vi "Write_Stats_Impedance_Meas.vi"(4 "Z Phase":dbl[](array[numeric]), 5 "|Z| Mag":dbl[](array[numeric]), 6 "Output Stats Cluster":T1, 7 "Compensation and Gain":T2={"Rg_Vmon"=5000.0, "Rg_Imon"=5000.0, "ESL_Cal"=2.5e-07, "ESR_Cal"=0.0, "Cp_Cal"=0.0, "Rp_Cal"=0.0, "Use Open/Short\nCompensation"=FALSE, "R_Shunt"=10000.0, "RLoad"=1000000000.0, "RLoad_Meas"=1000000000.0} {"RLoad_Meas" format="%#_6p"; "RLoad" format="%#_6p"}, 8 "Test Params Cluster":T3={"Test Freq. (Hz)"=0.0, "Output Signal Amplitude\nVolts Pk"=0.0, "Sampling Time (s)"=0.0, "Sampling Rate (Hz)"=0.0, "Output Channel"="Dev2/ao0", "Current Channel"="Dev2/ai0", "Voltage Channel"="Dev2/ai0", "Trigger Channel"="/Dev2/ao/StartTrigger", "Number of runs"=5}, 9 "Experiment Title":string="Experiment Title", 10 "File Name String":string="Test", 11 "Path":path=path "C:/Users/MPI/Documents/Test Saving Data") -> ()   [LabVIEW 2022 SP3]
panel:
  in  "Meta-Data Array":dbl[](array[numeric])=[1.0]
  out "TDMS path":path=path "C:/Users/MPI/Documents/Test Saving Data/2022_01_06_23_07_06_Test.tdms"
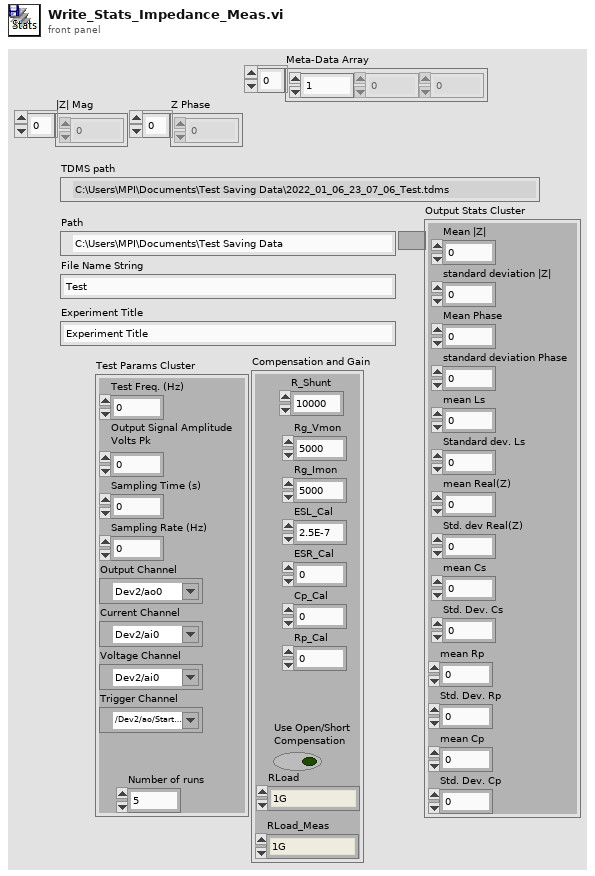
[diagram p1: front panel]
types:
  T1 = cluster{"Mean |Z|":dbl, "standard deviation |Z|":dbl, "Mean Phase":dbl, "standard deviation Phase":dbl, "mean Ls":dbl, "Standard dev. Ls":dbl, "mean Real(Z)":dbl, "Std. dev Real(Z)":dbl, "mean Cs":dbl, "Std. Dev. Cs":dbl, "Std. Dev. Rp":dbl, "mean Rp":dbl, "Std. Dev. Cp":dbl, "mean Cp":dbl}
  T2 = cluster{"Rg_Vmon":dbl, "Rg_Imon":dbl, "ESL_Cal":dbl, "ESR_Cal":dbl, "Cp_Cal":dbl, "Rp_Cal":dbl, "Use Open/Short\nCompensation":bool, "R_Shunt":dbl, "RLoad":dbl, "RLoad_Meas":dbl}
  T3 = cluster{"Test Freq. (Hz)":dbl, "Output Signal Amplitude\nVolts Pk":dbl, "Sampling Time (s)":dbl, "Sampling Rate (Hz)":dbl, "Output Channel":tag, "Current Channel":tag, "Voltage Channel":tag, "Trigger Channel":tag, "Number of runs":i32}
  T4 = enum16{"open", "open or create", "create or replace", "create", "open (read-only)"}
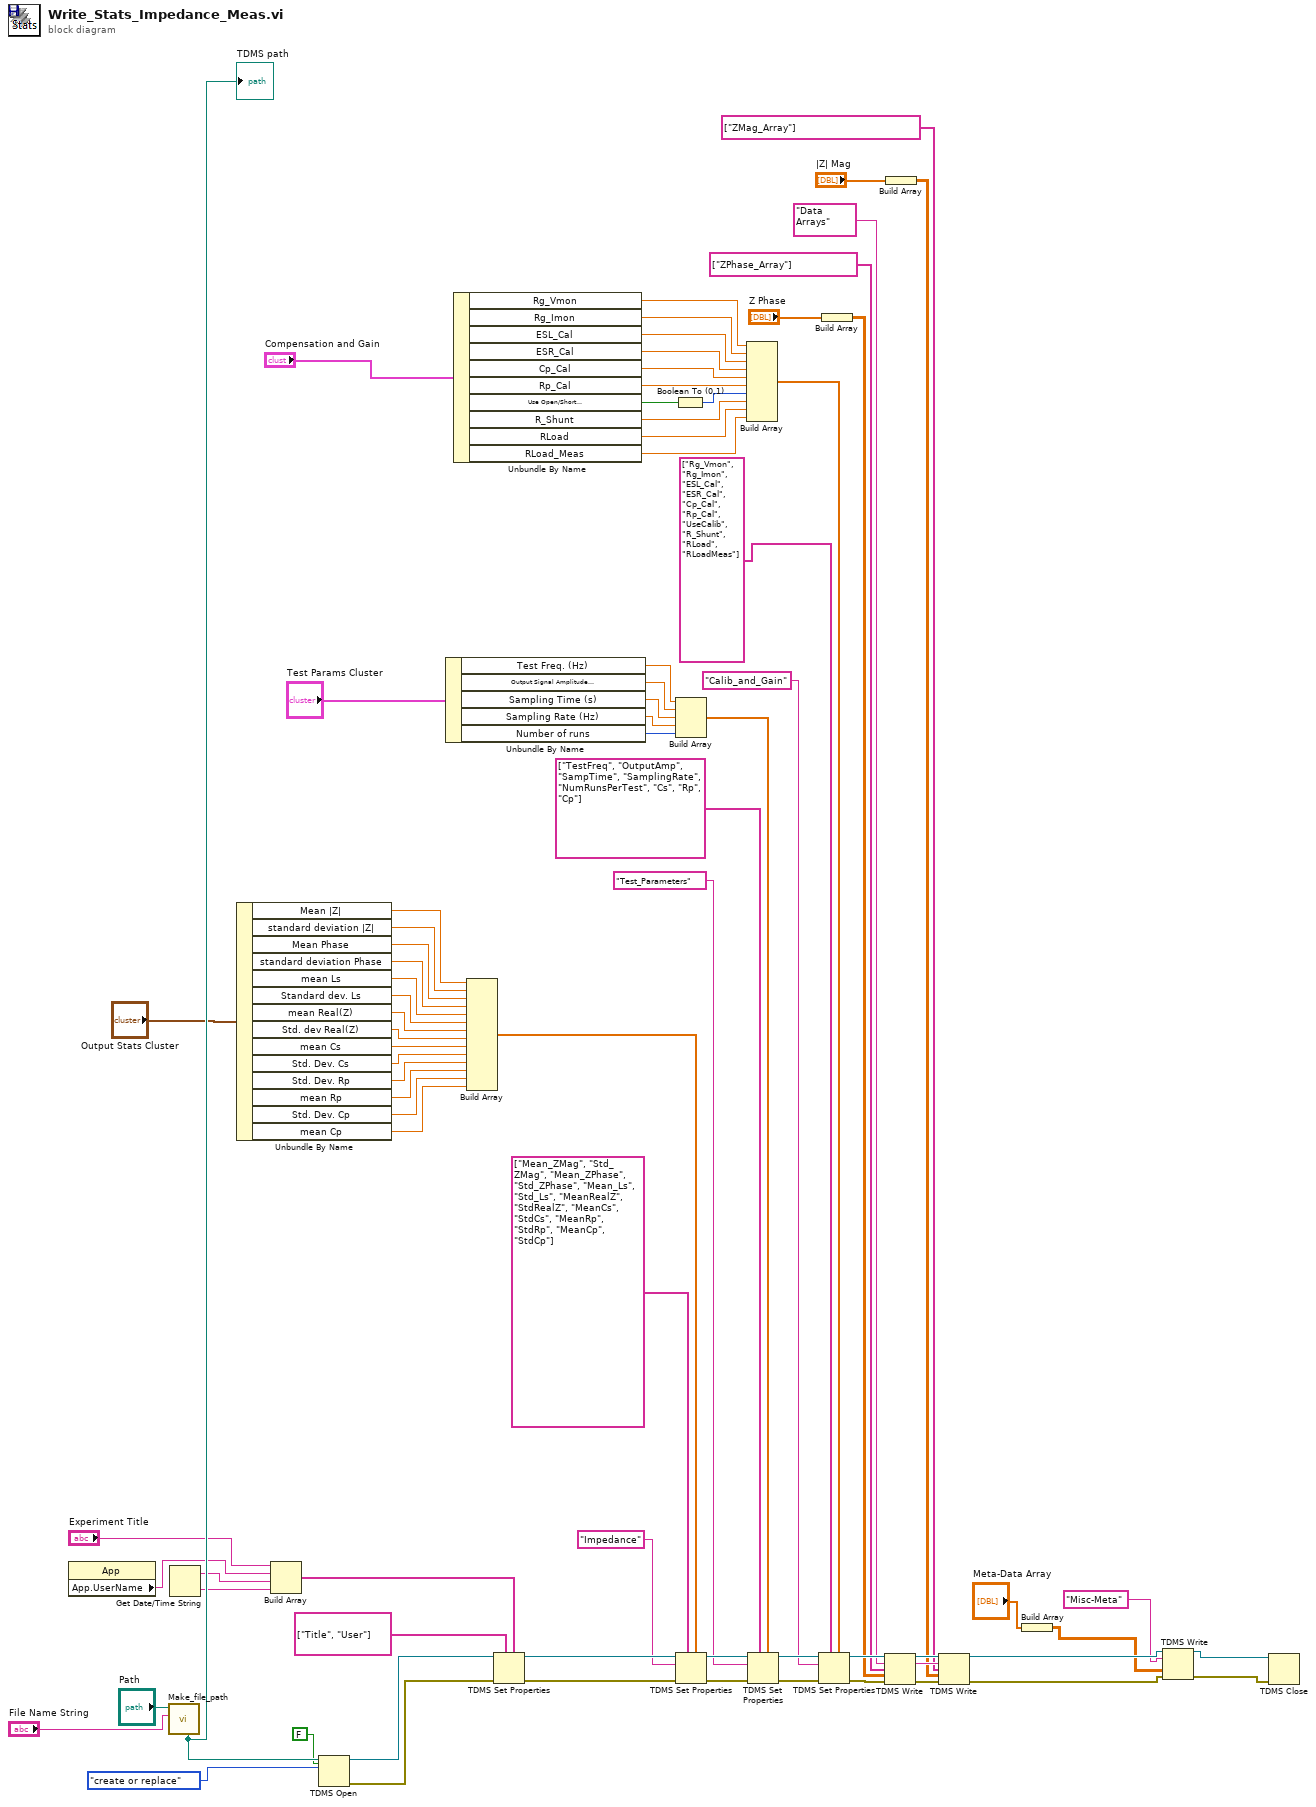
[diagram p0: block diagram]
diagram:
  n1 = property class="App"() -> ("App.UserName"=w75:string)  [unwired: 2 in, 2 out]
  n2 = call "Make_file_path.vi"("File Name String"="File Name String", "Base path"="Path") -> ("TDMS path"=w80:path)  [unwired: 9 in]
  "TDMS path" <- w80
  n3 = Get Date/Time String() -> (date string=w63:string, time string=w62:string)  [unwired: 3 in]
  n4 = Unbundle By Name("Output Stats Cluster") -> ("Mean |Z|"=w68:dbl, "standard deviation |Z|"=w66:dbl, "Mean Phase"=w65:dbl, "standard deviation Phase"=w64:dbl, "mean Ls"=w20:dbl, "Standard dev. Ls"=w19:dbl, "mean Real(Z)"=w18:dbl, "Std. dev Real(Z)"=w17:dbl, "mean Cs"=w16:dbl, "Std. Dev. Cs"=w15:dbl, "Std. Dev. Rp"=w14:dbl, "mean Rp"=w13:dbl, "Std. Dev. Cp"=w12:dbl, "mean Cp"=w11:dbl)
  n5 = Build Array("Experiment Title", w75, w63, w62) -> (w74:string[])
  n6 = TDMS Open(5:FALSE ("create index file? (T)"), 10:T4."create or replace" ("operation (0:open)"), 11:w80) -> (0:w34:errorcluster, 3:w72:refnum<k34>)  [unwired: 4 in]
  n7 = Unbundle By Name("Test Params Cluster") -> ("Test Freq. (Hz)"=w54:dbl, "Output Signal Amplitude\nVolts Pk"=w55:dbl, "Sampling Time (s)"=w56:dbl, "Sampling Rate (Hz)"=w57:dbl, "Number of runs"=w22:i32)
  n8 = Unbundle By Name("Compensation and Gain") -> ("Rg_Vmon"=w48:dbl, "Rg_Imon"=w47:dbl, "ESL_Cal"=w46:dbl, "ESR_Cal"=w45:dbl, "Cp_Cal"=w44:dbl, "Rp_Cal"=w43:dbl, "Use Open/Short\nCompensation"=w42:bool, "R_Shunt"=w39:dbl, "RLoad"=w2:dbl, "RLoad_Meas"=w1:dbl)
  n9 = Build Array(w68, w66, w65, w64, w20, w19, w18, w17, w16, w15, w14, w13, w12, w11) -> (w69:dbl[])
  n10 = TDMS Set Properties(5:w74, 7:string[] ["Title", "User"] ("property names"), 8:w34, 11:w72) -> (0:w33:errorcluster, 3:w71:refnum<k34>)  [unwired: 4 out]
  n11 = Boolean To (0,1)(Boolean=w42) -> (0, 1=w41:i16)
  n12 = Build Array(w54, w55, w56, w57, w22) -> (w53:dbl[])
  n13 = TDMS Set Properties(5:w69, 7:string[] ["Mean_ZMag", "Std_ZMag", "Mean_ZPhase", "Std_ZPhase", "Mean_Ls", "Std_Ls", "MeanRealZ", "StdRealZ", "MeanCs", "StdCs", "MeanRp", "StdRp", "MeanCp", "StdCp"] ("property names"), 8:w33, 10:"Impedance" ("group name"), 11:w71) -> (0:w32:errorcluster, 3:w59:refnum<k34>)  [unwired: 3 out]
  n14 = Build Array(w48, w47, w46, w45, w44, w43, w41, w39, w2, w1) -> (w40:dbl[])
  n15 = TDMS Set Properties(5:w53, 7:string[] ["TestFreq", "OutputAmp", "SampTime", "SamplingRate", "NumRunsPerTest", "Cs", "Rp", "Cp"] ("property names"), 8:w32, 10:"Test_Parameters" ("group name"), 11:w59) -> (0:w31:errorcluster, 3:w50:refnum<k34>)  [unwired: 3 out]
  n16 = TDMS Set Properties(5:w40, 7:string[] ["Rg_Vmon", "Rg_Imon", "ESL_Cal", "ESR_Cal", "Cp_Cal", "Rp_Cal", "UseCalib", "R_Shunt", "RLoad", "RLoadMeas"] ("property names"), 8:w31, 10:"Calib_and_Gain" ("group name"), 11:w50) -> (0:w30:errorcluster, 3:w38:refnum<k34>)  [unwired: 3 out]
  n17 = Build Array("Z Phase") -> (w27:dbl[][])
  n18 = TDMS Write(0:w38, 5:"Data Arrays" ("group name"), 7:string[] ["ZPhase_Array"] ("channel name(s) in (Untitled)"), 9:w27, 11:w30) -> (4:w37:refnum<k34>, 6:w35:string, 15:w29:errorcluster)  [unwired: 1 in, 1 out]
  n19 = Build Array("|Z| Mag") -> (w25:dbl[][])
  n20 = TDMS Write(0:w37, 5:w35, 7:string[] ["ZMag_Array"] ("channel name(s) in (Untitled)"), 9:w25, 11:w29) -> (4:w8:refnum<k34>, 15:w7:errorcluster)  [unwired: 1 in, 2 out]
  n21 = Build Array("Meta-Data Array") -> (w4:dbl[][])
  n22 = TDMS Write(0:w8, 5:"Misc-Meta" ("group name in (Untitled)"), 9:w4, 11:w7) -> (4:w9:refnum<k34>, 15:w6:errorcluster)  [unwired: 2 in, 2 out]
  n23 = TDMS Close(8:w6, 11:w9) -> ()  [unwired: 2 out]
